vi "DeQueueMain.vi"(0 "object in":refnum<class "Application.lvclass">=refnum, 2 "timeout in ms (-1)":i32=-1, 5 "error in (no error)":errorcluster) -> (14 "object out":refnum<class "Application.lvclass">, 16 "Message":string, 17 "Message Data":variant=variant(errorcluster {"status"=TRUE, "code"=1, "source"="MainTemplate.vi<ERR>\nThe invalid message string \"\" was received in the Message Handling Loop.\n\n\n<b>Complete call chain:</b>\r\n     MainTemplate.vi"}), 19 "error out":errorcluster)   [LabVIEW 2021, in "Application.lvclass"]
uses:
  Application.lvclass
  CetoniPump_class/CetoniPump.lvclass
  AD2_SDK_class/AD2_SDK.lvclass
  Hamamatsu_class/Hamamatsu.lvclass
  Application.lvclass/Application.ctl
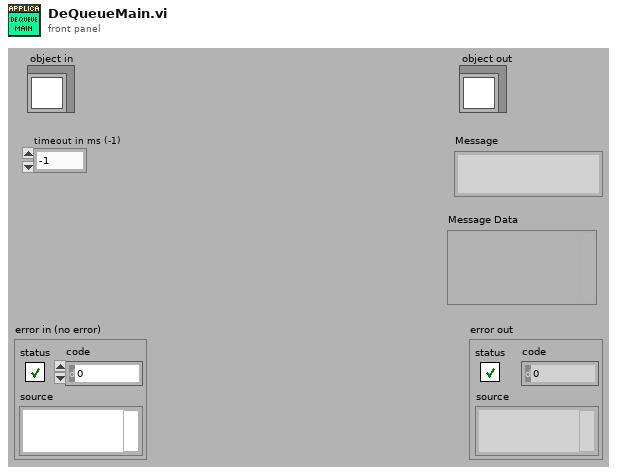
[diagram p1: front panel]
types:
  T1 = cluster{"Message":string, "Message Data":variant}
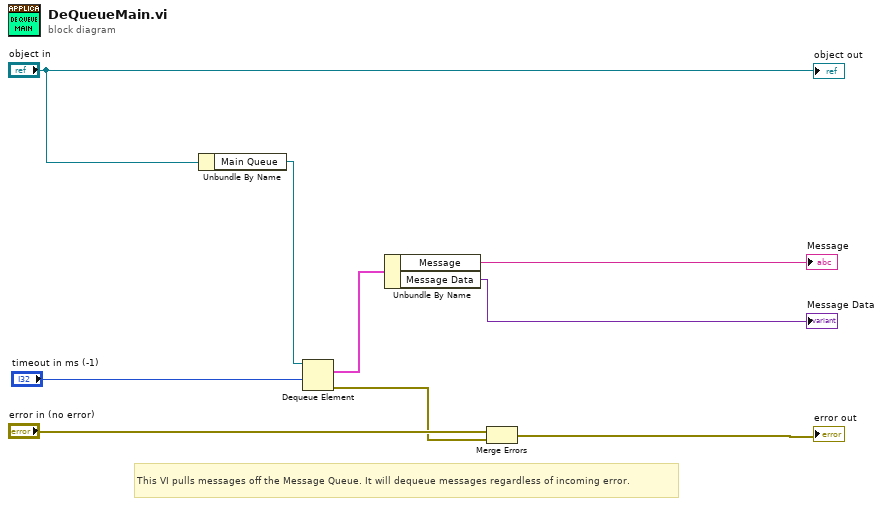
[diagram p0: block diagram]
diagram:
  # "This VI pulls messages off the Message Queue. It will dequeue messages regardless of incoming error."
  n1 = Unbundle By Name("object in") -> ("Main Queue"=w1:refnum<queue>)
  n2 = Dequeue Element(queue=w1, timeout in ms (-1)="timeout in ms (-1)") -> (element=w3:T1, error out=w2:errorcluster)  [unwired: 1 in, 2 out]
  n3 = Unbundle By Name(w3) -> ("Message"=→"Message":string, "Message Data"=→"Message Data":variant)
  n4 = Merge Errors("error in (no error)", w2) -> (→"error out":errorcluster)
  "object out" <- "object in"
